vi "Start Time to Minutes.vi"(8 "error in (no error)":errorcluster, 11 "Start Time":string="8:30") -> (0 "error out":errorcluster, 3 "Minutes":i32)   [LabVIEW 2026]
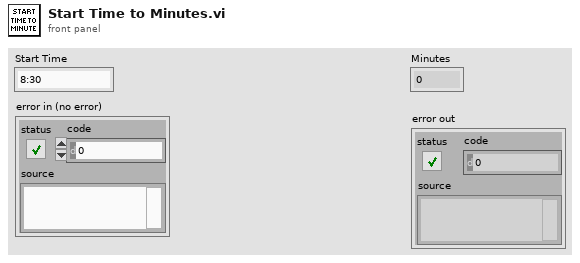
[diagram p1: front panel]
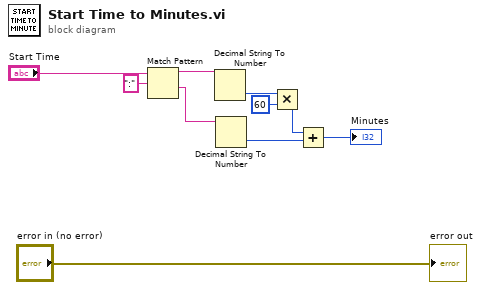
[diagram p0: block diagram]
diagram:
  n1 = Match Pattern(string="Start Time", regular expression=":") -> (before substring=w5:string, after substring=w8:string)  [unwired: 1 in, 2 out]
  n2 = Decimal String To Number(string=w5) -> (number=w6:i32)  [unwired: 2 in, 1 out]
  n3 = Decimal String To Number(string=w8) -> (number=w10:i32)  [unwired: 2 in, 1 out]
  n4 = Multiply(x=w6, y=60) -> (x*y=w9:i32)
  n5 = Add(x=w9, y=w10) -> (x+y=→"Minutes":i32)
  "error out" <- "error in (no error)"
